vi "InitialConditionTest.vi"() -> ()   [LabVIEW 2016]
uses:
  Car Wash 16.0/Controls/Wash Options.ctl
  Car Wash 16.0/Controls/Car Wash Indicators.ctl
  Car Wash 16.0/Car Wash.vi
  main/apis/Setup/GetVI/GetVIByPath.vi
  main/apis/Assert/AssertControlValueCompare/AssertControlValueEqual.vi
  main/apis/Stimulus/ValueSignalByPathString.vi
  <vilib>/addons/_JKI Toolkits/Caraya/classes/Test/Test.lvclass
  Car Wash 16.0/Car Wash.lvlib
panel:
  out "error out":errorcluster
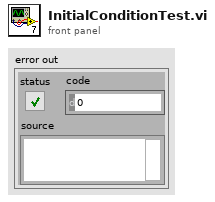
[diagram p1: front panel]
types:
  T1 = typedef "Car Wash.lvlib/Car Wash Indicators.ctl" = cluster{"Under Body Wash":bool, "Bug Remover":bool, "Pre-Soak":bool, "High Pressure Wash":bool, "Low Pressure Wax":bool, "Spot Free Rinse":bool, "Tire Shine Foam":bool, "Air Dry":bool, "Vehicle Out of Position":bool}
  T2 = typedef "Car Wash.lvlib/Wash Options.ctl" = cluster{"Underbody Wash":bool, "Bug Remover":bool, "Pre-Soak":bool, "High Pressure Wash":bool, "Low Pressure Wax":bool, "Spot Free Rinse":bool, "Tire Shine Foam":bool, "Air Dry":bool}
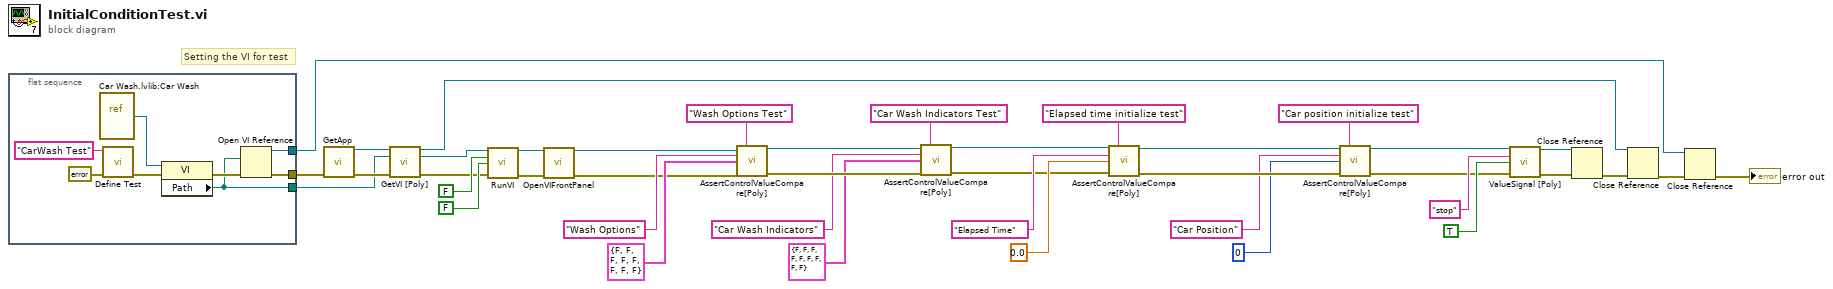
[diagram p0: block diagram]
diagram:
  # "Setting the VI for test"
  n1 = flat-sequence {
    tunnel: [w45] -> w23
    tunnel: [w44] -> w1
    tunnel: [w42] -> w18
    frame #0 {
      n2 = vi-ref "Car Wash.lvlib:Car Wash.vi"() -> (w47:refnum<vi>)
      n3 = call <vilib>:"Define Test.vi"("error in (no error)"=errorcluster {"status"=FALSE, "code"=0, "source"=""}, "Label (VI Title)"="CarWash Test") -> ("error out"=w48:errorcluster)  [unwired: 9 in]
      n4 = property on="Property Node" class="VI"(reference=w47, error in=w48) -> (error out=w46:errorcluster, "Path"=w42:path)  [unwired: 1 out]
      n5 = Open VI Reference(vi path=w42, error in (no error)=w46) -> (vi reference=w44:refnum<vi>, error out=w45:errorcluster)  [unwired: 4 in]
    }
  }
  n6 = call "GetApp.vi"("error in (no error)"=w23) -> ("Application Ref"=w19:refnum<vi>, "error out"=w20:errorcluster)  [unwired: 13 in]
  n7 = call-poly "GetVI [Poly].vi"("Application Ref in"=w19, "VI Path"=w18, "error in (no error)"=w20) -> ("Application Ref out"=w2:refnum<vi>, "VI Reference"=w17:refnum<vi>, "error out"=w16:errorcluster)  [unwired: 10 in]
  n8 = call "RunVI.vi"("VI Reference In"=w17, "Wait Until Done (F)"=FALSE ("Wait Until Done"), "Auto Dispose Reference (F)"=FALSE ("Auto Dispose Reference"), "error in"=w16) -> ("VI Reference Out"=w14:refnum<vi>, "error out"=w15:errorcluster)  [unwired: 10 in]
  n9 = call "OpenVIFrontPanel.vi"("VI Reference In"=w14, "error in"=w15) -> ("VI Reference Out"=w3:refnum<vi>, "error out"=w13:errorcluster)  [unwired: 12 in]
  n10 = call-poly "AssertControlValueCompare[Poly].vi"("VI Reference In"=w3, "Label"="Wash Options Test", "Control Name"="Wash Options", "Control Value"=T2 {"Underbody Wash"=FALSE, "Bug Remover"=FALSE, "Pre-Soak"=FALSE, "High Pressure Wash"=FALSE, "Low Pressure Wax"=FALSE, "Spot Free Rinse"=FALSE, "Tire Shine Foam"=FALSE, "Air Dry"=FALSE} ("Wash Options"), "error out"=w13) -> ("VI Reference Out"=w27:refnum<vi>, "error out"=w30:errorcluster)  [unwired: 9 in]
  n11 = call-poly "AssertControlValueCompare[Poly].vi"("VI Reference In"=w27, "Label"="Car Wash Indicators Test", "Control Name"="Car Wash Indicators", "Control Value"=T1 {"Under Body Wash"=FALSE, "Bug Remover"=FALSE, "Pre-Soak"=FALSE, "High Pressure Wash"=FALSE, "Low Pressure Wax"=FALSE, "Spot Free Rinse"=FALSE, "Tire Shine Foam"=FALSE, "Air Dry"=FALSE, "Vehicle Out of Position"=FALSE} ("Car Wash Indicators"), "error out"=w30) -> ("VI Reference Out"=w28:refnum<vi>, "error out"=w29:errorcluster)  [unwired: 9 in]
  n12 = call-poly "AssertControlValueCompare[Poly].vi"("VI Reference In"=w28, "Label"="Elapsed time initialize test", "Control Name"="Elapsed Time", "Control Value"=0.0, "error out"=w29) -> ("VI Reference Out"=w36:refnum<vi>, "error out"=w37:errorcluster)  [unwired: 9 in]
  n13 = call-poly "AssertControlValueCompare[Poly].vi"("VI Reference In"=w36, "Label"="Car position initialize test", "Control Name"="Car Position", "Control Value"=u8 0, "error out"=w37) -> ("VI Reference Out"=w4:refnum<vi>, "error out"=w5:errorcluster)  [unwired: 9 in]
  n14 = call-poly "ValueSignal [Poly].vi"("VI Reference In"=w4, "Control Name"="stop", "Value (Signaling)"=TRUE, "error in"=w5) -> ("VI Reference Out"=w8:refnum<vi>, "error out"=w10:errorcluster)  [unwired: 10 in]
  n15 = Close Reference(reference=w8, error in (no error)=w10) -> (error out=w9:errorcluster)
  n16 = Close Reference(reference=w2, error in (no error)=w9) -> (error out=w7:errorcluster)
  n17 = Close Reference(reference=w1, error in (no error)=w7) -> (error out=→"error out":errorcluster)
